vi "Byte Buffer.Mapping.Create (Data Reference).vi"(8 "error in (no error)":errorcluster, 9 "data type":T1, 10 "buffer offset":i32, 11 "Data Reference":T2 format="%.0x") -> (0 "error out":errorcluster, 2 "new buffer offset":i32, 3 "mapping":T3)   [LabVIEW 2016, in "VeriStand Data.lvlib" / "Byte Buffer.lvclass"]
uses:
  Byte Buffer.lvclass
  Byte Buffer.Mapping.ctl
  Typedefs/Typedefs.Data Types.ctl
  <vilib>/NI Veristand/Custom Device API/Data Reference.ctl
  Data Channels/Channels.Inline.Reference Error Handler.vi
  Utilities/Utilities.Sizeof.Scalar.vi
  <vilib>/NI Veristand/Custom Device API/Global Data Refs.vi
  VeriStand Data.lvlib
  <vilib>/NI Veristand/Custom Device API/Custom Device API.lvlib
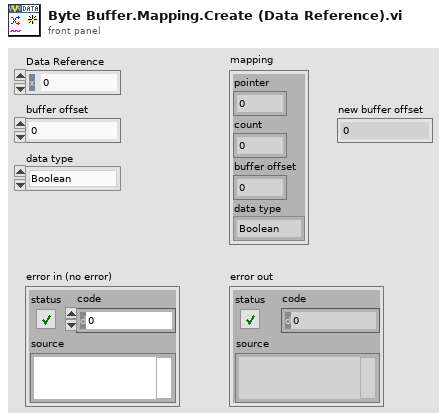
[diagram p1: front panel]
types:
  T1 = typedef "VeriStand Data.lvlib/Typedefs.Data Types.ctl" = enum16{"Boolean", "Single", "Double", "I8", "I16", "I32", "I64", "U8", "U16", "U32", "U64"}
  T2 = typedef "Custom Device API.lvlib/Data Reference.ctl" = i32
  T3 = typedef "VeriStand Data.lvlib/Byte Buffer.lvclass/Byte Buffer.Mapping.ctl" = cluster{"pointer":u64, "count":i32, "buffer offset":i32, "data type":T1}
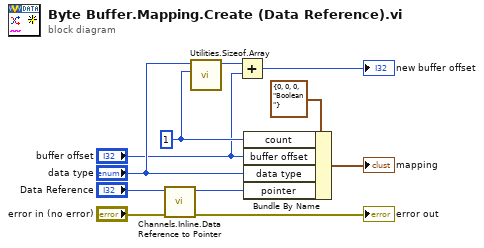
[diagram p0: block diagram]
diagram:
  w4 = 1 ("count")
  n1 = call "Channels.Inline.Data Reference to Pointer.vi"("error in (no error)"="error in (no error)", "Data Reference in"="Data Reference") -> ("error out"=→"error out":errorcluster, "Channel Pointer"=w8:u64)  [unwired: 8 in]
  n2 = call "Utilities.Sizeof.Array.vi"("count"=w4, "data type"="data type") -> ("size"=w3:i32)  [unwired: 9 in]
  n3 = Add(x=w3, y="buffer offset") -> (x+y=→"new buffer offset":i32)
  n4 = Bundle By Name(cluster=T3 {"pointer"=0, "count"=0, "buffer offset"=0, "data type"=enum."Boolean"} ("mapping"), "count"=w4, "buffer offset"="buffer offset", "data type"="data type", "pointer"=w8) -> (→"mapping":T3)
